vi "Write Publish Analyze Results Msg.vi"(8 "error in (no error)":errorcluster, 10 "Publish Analyze Results Msg.lvclass":refnum<class "Publish Analyze Results Msg.lvclass">, 11 "HIJ Single Cam App Demo in":refnum<class "HIJ Vision Camera App w Timer.lvclass">) -> (0 "error out":errorcluster, 3 "HIJ Single Cam App Demo out":refnum<class "HIJ Vision Camera App w Timer.lvclass">)   [LabVIEW 2014, in "HIJ Vision Camera App w Timer.lvlib" / "HIJ Vision Camera App w Timer.lvclass"]
uses:
  HIJ Vision Camera App w Timer.lvclass
  Abstract Messages/Publish Analyze Results Msg/Publish Analyze Results Msg.lvclass
  HIJ Vision Camera App w Timer.lvclass/HIJ Vision Camera App w Timer.ctl
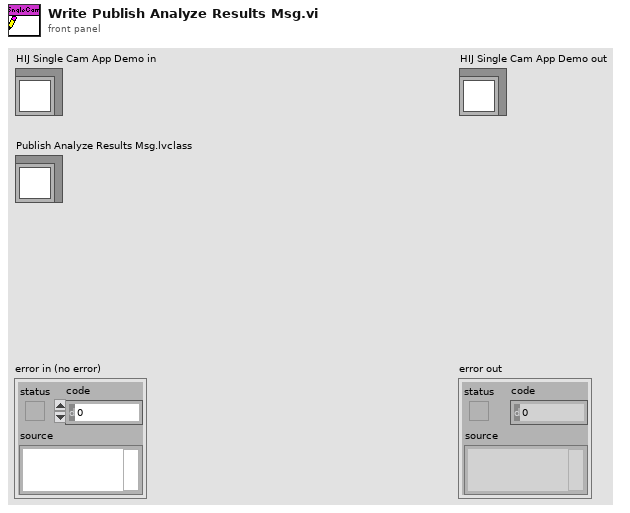
[diagram p1: front panel]
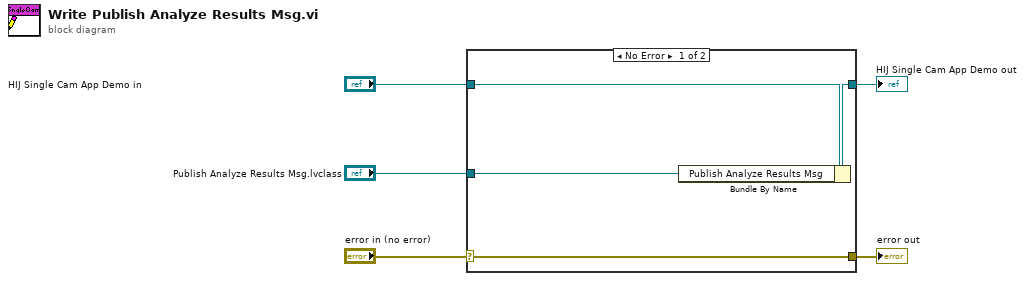
[diagram p0: block diagram]
diagram:
  n1 = case shown="No Error" "error in (no error)" {
    selector: "error in (no error)" -> [w9 w10]
    tunnel: [w9 w10] -> w4
    tunnel: [w7 w11] -> w2
    tunnel: "HIJ Single Cam App Demo in" -> [w8 w11]
    tunnel: "Publish Analyze Results Msg.lvclass" -> [w6 _]
    frame No Error {
      n2 = Bundle By Name(cluster=w8, "Publish Analyze Results Msg"=w6) -> (w7:refnum<class "HIJ Vision Camera App w Timer.lvclass">)
    }
    frame Error {
    }
  }
  "error out" <- w4
  "HIJ Single Cam App Demo out" <- w2
